vi "CMN_Cali.vi"(11 "Enum":T1(ring)=enum."CF_Z_Bridge") -> ()   [LabVIEW 2013]
uses:
  <vilib>/Utility/file.llb/Write To Spreadsheet File (DBL).vi
panel:
  out "C1":dbl
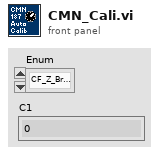
[diagram p1: front panel]
types:
  T1 = enum16{"CF", "CF_Z_Bridge", "MNK", "MNK_Z_Bridge"}
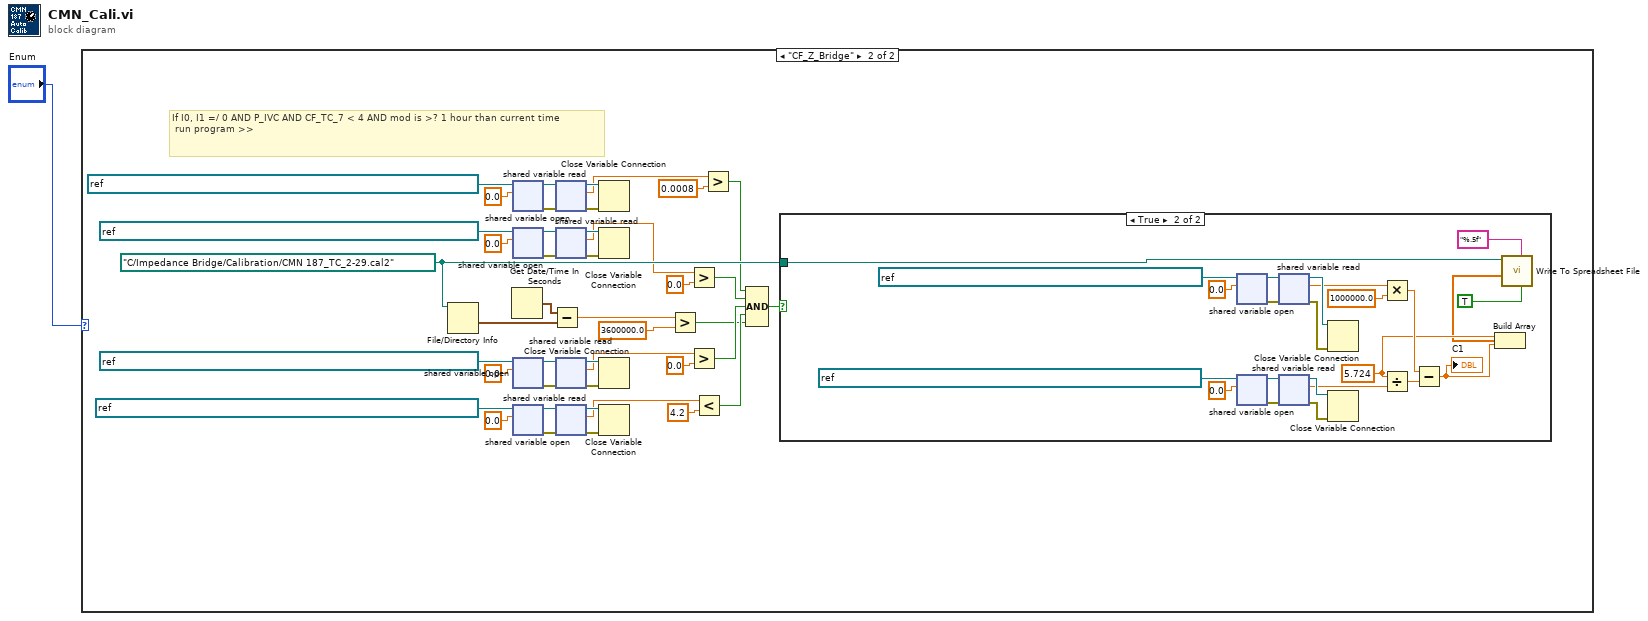
[diagram p0: block diagram]
diagram:
  n1 = case shown="\"CF_Z_Bridge\"" "Enum" {
    frame "CF", Default {
    }
    frame "CF_Z_Bridge" {
      w44 = path "C:/Impedance Bridge/Calibration/CMN 187_TC_2-29.cal2" ("file path (dialog if empty)")
      # "If I0, I1 =/ 0 AND P_IVC AND CF_TC_7 < 4 AND mod is >? 1 hour than current time\n run program >>"
      n2 = File/Directory Info(path=w44) -> (last mod=w5:timestamp)  [unwired: 1 in, 6 out]
      n3 = Get Date/Time In Seconds() -> (seconds since 1Jan1904=w6:timestamp)
      n4 = shared-variable-open(refnum<k21> "ni.var.psp://housesoftheholy/Leiden CF900/Leiden CF FP/CF FP MG3" ("shared variable refnum in"), 0.0 ("y")) -> (w27:refnum<k21>, w25:errorcluster)  [unwired: 2 in]
      n5 = shared-variable-open(refnum<k21> "ni.var.psp://housesoftheholy/Leiden CF900/Leiden CF TC/CF TC I0" ("shared variable refnum in"), 0.0 ("y")) -> (w43:refnum<k21>, w41:errorcluster)  [unwired: 2 in]
      n6 = shared-variable-open(refnum<k21> "ni.var.psp://housesoftheholy/Leiden CF900/Leiden CF TC/CF TC I1" ("shared variable refnum in"), 0.0 ("y")) -> (w37:refnum<k21>, w35:errorcluster)  [unwired: 2 in]
      n7 = shared-variable-open(refnum<k21> "ni.var.psp://housesoftheholy/Leiden CF900/Leiden CF TC/CF TC T7" ("shared variable refnum in"), 0.0 ("y")) -> (w10:refnum<k21>, w12:errorcluster)  [unwired: 2 in]
      n8 = Subtract(x=w6, y=w5) -> (x-y=w4:dbl)
      n9 = shared-variable-read(w27, w25) -> (w26:refnum<k21>, w24:errorcluster, w21:dbl)  [unwired: 1 out]
      n10 = shared-variable-read(w43, w41) -> (w42:refnum<k21>, w40:errorcluster, w31:dbl)  [unwired: 1 out]
      n11 = shared-variable-read(w37, w35) -> (w36:refnum<k21>, w34:errorcluster, w28:dbl)  [unwired: 1 out]
      n12 = shared-variable-read(w10, w12) -> (w11:refnum<k21>, w13:errorcluster, w9:dbl)  [unwired: 1 out]
      n13 = Close Variable Connection(8:w24, 11:w26) -> ()  [unwired: 1 out]
      n14 = Close Variable Connection(8:w40, 11:w42) -> ()  [unwired: 1 out]
      n15 = Close Variable Connection(8:w34, 11:w36) -> ()  [unwired: 1 out]
      n16 = Close Variable Connection(8:w13, 11:w11) -> ()  [unwired: 1 out]
      n17 = Greater?(x=w4, y=3600000.0) -> (0:w2:bool)
      n18 = Greater?(x=w31, y=0.0) -> (0:w18:bool)
      n19 = Greater?(x=w28, y=0.0) -> (0:w17:bool)
      n20 = Less?(x=w9, y=4.2) -> (x < y?=w7:bool)
      n21 = Greater?(x=w21, y=0.0008) -> (0:w19:bool)
      n22 = Compound Arithmetic op=AND(w19, w18, w17, w7, w2) -> (w16:bool)
      n23 = case shown="True" w16 {
        tunnel: w44 -> [_ w45]
        frame False {
        }
        frame True {
          w64 = 5.724 ("x")
          n24 = shared-variable-open(refnum<k21> "ni.var.psp://housesoftheholy/Leiden CF900/CF_TC_Z_R0" ("shared variable refnum in"), 0.0 ("y")) -> (w59:refnum<k21>, w57:errorcluster)  [unwired: 2 in]
          n25 = shared-variable-open(refnum<k21> "ni.var.psp://housesoftheholy/Leiden CF900/Leiden CF TC/CF TC T7" ("shared variable refnum in"), 0.0 ("y")) -> (w47:refnum<k21>, w49:errorcluster)  [unwired: 2 in]
          n26 = shared-variable-read(w59, w57) -> (w58:refnum<k21>, w56:errorcluster, w53:dbl)  [unwired: 1 out]
          n27 = shared-variable-read(w47, w49) -> (w48:refnum<k21>, w50:errorcluster, w46:dbl)  [unwired: 1 out]
          n28 = Close Variable Connection(8:w56, 11:w58) -> ()  [unwired: 1 out]
          n29 = Close Variable Connection(8:w50, 11:w48) -> ()  [unwired: 1 out]
          n30 = Multiply(x=w53, y=1000000.0) -> (x*y=w65:dbl)
          n31 = Divide(x=w64, y=w46) -> (x/y=w67:dbl)
          n32 = Subtract(x=w65, y=w67) -> (x-y=w63:dbl)
          "C1" <- w63
          n33 = Build Array(w64, w63) -> (w62:dbl[])
          n34 = call-poly <vilib>:"Write To Spreadsheet File.vi"("transpose? (no:F)"=TRUE, "format (%.3f)"="%.5f", "1D data"=w62, "file path (dialog if empty)"=w45) -> ()  [unwired: 4 in, 1 out]
        }
      }
    }
  }
